vi "Apply Amplitude Envelope.vi"(5 "profile":enum16{"Linear", "Half cosine"}(ring), 6 "time elapsed at transition":dbl, 8 "error in (no error)":errorcluster, 9 "duration":dbl=-1.0, 10 "amplitude modulation":cluster{"start":dbl, "stop":dbl}={"start"=1.0, "stop"=1.0}, 11 "waveform in":waveform(dbl)={"t0"=timestamp(0 s since 1904-01-01), "dt"=0.1, "Y"=[1.0, 1.0, 1.0, 1.0, 1.0]}) -> (0 "error out":errorcluster, 2 "amplitude envelope last value":dbl, 3 "waveform out":waveform(dbl)={"t0"=timestamp(0 s since 1904-01-01), "dt"=nan, "Y"=[]})   [LabVIEW 2017, in "SV Signal.lvclass"]
uses:
  <vilib>/addons/_NISVFA/_Generation/Signal Generation/SV Signal/SV Signal.lvclass
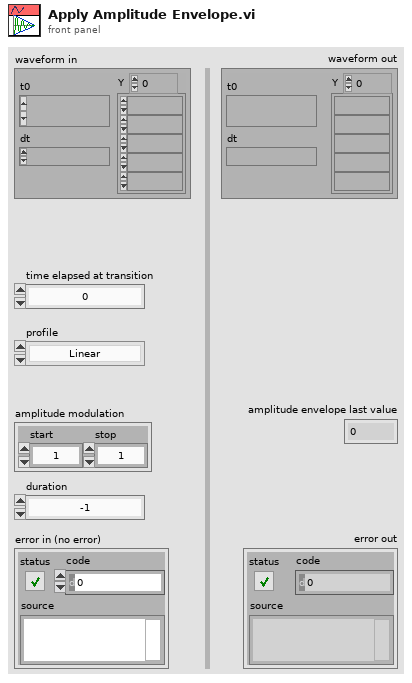
[diagram p1: front panel]
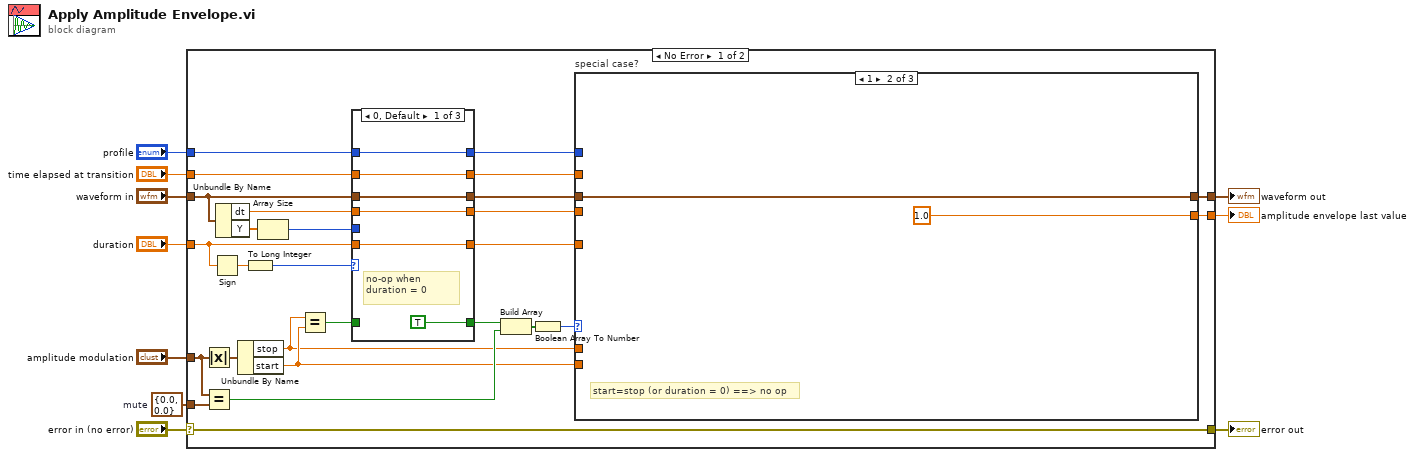
[diagram p0: block diagram]
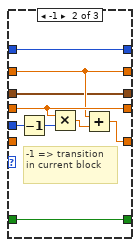
[diagram p2: hidden frame]
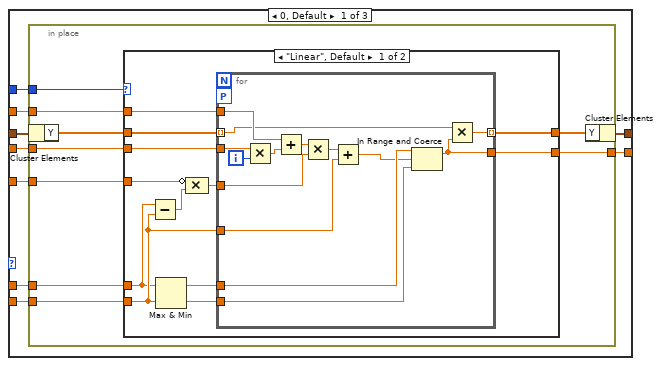
[diagram p4: hidden frame]
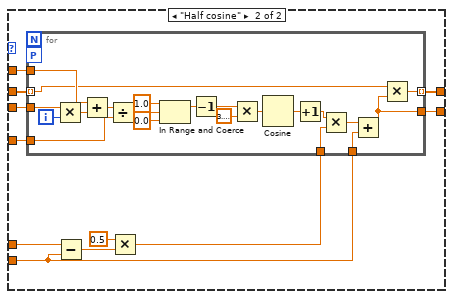
[diagram p5: hidden frame]
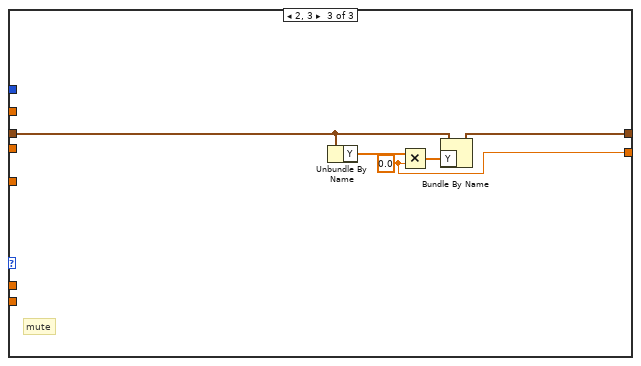
[diagram p6: hidden frame]
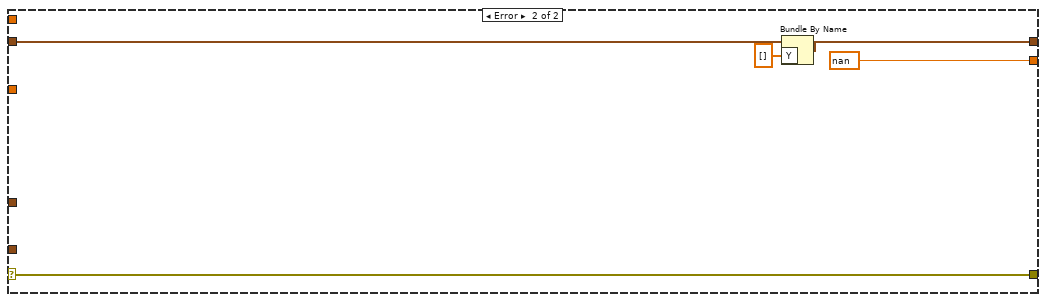
[diagram p7: hidden frame]
diagram:
  w6 = cluster{"start":dbl, "stop":dbl} {"start"=0.0, "stop"=0.0}  # mute
  n1 = case shown="No Error" "error in (no error)" {
    selector: "error in (no error)" -> [w13 w144]
    tunnel: "amplitude modulation" -> [w37 _]
    tunnel: [w36 nan ("start")] -> w9
    tunnel: "time elapsed at transition" -> [w22 _]
    tunnel: "profile" -> [w24 _]
    tunnel: w6 -> [w29 _]
    tunnel: "duration" -> [w19 _]
    tunnel: [w28 w142] -> w4
    tunnel: "waveform in" -> [w18 w143]
    tunnel: [w13 w144] -> w1
    frame No Error {
      n2 = Absolute Value(x=w37) -> (abs(x)=w30:cluster{"start":dbl, "stop":dbl})
      n3 = Equal?(x=w37, y=w29) -> (x = y?=w33:bool)
      n4 = Sign(1:w19) -> (0:w27:dbl)
      n5 = Unbundle By Name(w18) -> ("dt"=w15:dbl, "Y"=w17:dbl[])
      n6 = Unbundle By Name(w30) -> ("stop"=w31:dbl, "start"=w32:dbl)
      n7 = To Long Integer(number=w27) -> (32bit integer=w26:i32)
      n8 = Array Size(array=w17) -> (size(s)=w16:i32)
      n9 = Equal?(x=w31, y=w32) -> (x = y?=w12:bool)
      n10 = case shown="0, Default" w26 {
        tunnel: [w43 w52 w58] -> w25
        tunnel: w24 -> [w43 w52 w58]
        tunnel: [w42 w49 w57] -> w23
        tunnel: w22 -> [w42 w49 w57]
        tunnel: [w41 w46 w56] -> w21
        tunnel: w18 -> [w41 w46 w56]
        tunnel: [w40 w47 w55] -> w20
        tunnel: w19 -> [w40 _ w55]
        tunnel: w16 -> [_ w51 _]
        tunnel: w15 -> [w39 w50 w54]
        tunnel: [w39 w50 w54] -> w14
        tunnel: w12 -> [_ w44 w53]
        tunnel: [TRUE w44 w53] -> w11
        frame 0, Default {
          # "no-op when duration = 0"
        }
        frame -1 {
          # "-1 => transition in current block"
          n11 = Decrement(x=w51) -> (x-1=w45:i32)
          n12 = Multiply(x=w50, y=w45) -> (x*y=w48:dbl)
          n13 = Add(x=w49, y=w48) -> (x+y=w47:dbl)
        }
        frame 1 {
        }
      }
      n14 = Build Array(w11, w33) -> (w34:bool[])
      n15 = Boolean Array To Number(Boolean array=w34) -> (number=w35:u32)
      n16 = case "special case?" shown="1" w35 {
        tunnel: w21 -> [w67 w136 w138]
        tunnel: [w66 w136 w141] -> w28
        tunnel: w20 -> [w65 _ _]
        tunnel: w31 -> [w62 _ _]
        tunnel: w32 -> [w61 _ _]
        tunnel: w25 -> [w64 _ _]
        tunnel: w23 -> [w63 _ _]
        tunnel: w14 -> [w60 _ _]
        tunnel: [w59 1.0 ("t") w137] -> w36
        frame 0, Default {
          n17 = in-place {
            in-place-border: w63 -> [w74]
            in-place-border: w64 -> [w70]
            in-place-border: w65 -> [w73]
            in-place-border: w62 -> [w69]
            in-place-border: w61 -> [w68]
            in-place-border: w60 -> [w72]
            in-place-border: [w71] -> w59
            n18 = in-place-cluster #1(w67) -> ("Y"=w76:dbl[])
            n19 = case shown="\"Linear\", Default" w70 {
              tunnel: w76 -> [w88 w113]
              tunnel: w72 -> [w87 w112]
              tunnel: w74 -> [w86 w107]
              tunnel: [w85 w111] -> w75
              tunnel: w73 -> [w81 w110]
              tunnel: w68 -> [w79 w104]
              tunnel: [w80 w106] -> w71
              tunnel: w69 -> [w78 w105]
              frame "Linear", Default {
                n20 = Subtract(x=w78, y=w79) -> (x-y=w77:dbl)
                n21 = Max & Min(x=w78, y=w79) -> (max(x,y)=w84:dbl, min(x,y)=w83:dbl)
                n22 = Compound Arithmetic op=MULTIPLY(invert w81, w77) -> (w82:dbl)
                n23 = for {
                  tunnel: w88 -> [w99] mode=indexing
                  tunnel: w87 -> [w102]
                  tunnel: w86 -> [w100]
                  tunnel: [w98] -> w85 mode=indexing
                  tunnel: w82 -> [w97]
                  tunnel: w79 -> [w95]
                  tunnel: w84 -> [w92]
                  tunnel: w83 -> [w91]
                  tunnel: [w90] -> w80
                  workers-P: _ -> [_]
                  i -> [w93]
                  n24 = Multiply(x=w102, y=w93) -> (x*y=w101:dbl)
                  n25 = Add(x=w100, y=w101) -> (x+y=w96:dbl)
                  n26 = Multiply(x=w96, y=w97) -> (x*y=w94:dbl)
                  n27 = Add(x=w94, y=w95) -> (x+y=w89:dbl)
                  n28 = In Range and Coerce(upper limit=w92, x=w89, lower limit=w91) -> (coerced(x)=w90:dbl)  [unwired: 1 out]
                  n29 = Multiply(x=w99, y=w90) -> (x*y=w98:dbl)
                }
              }
              frame "Half cosine" {
                n30 = Subtract(x=w105, y=w104) -> (x-y=w103:dbl)
                n31 = Multiply(x=0.5 ("y"), y=w103) -> (x*y=w108:dbl)
                n32 = for {
                  tunnel: w113 -> [w131] mode=indexing
                  tunnel: w112 -> [w134]
                  tunnel: w107 -> [w132]
                  tunnel: [w130] -> w111 mode=indexing
                  tunnel: w110 -> [w128]
                  tunnel: w108 -> [w117]
                  tunnel: w104 -> [w116]
                  tunnel: [w114] -> w106
                  workers-P: _ -> [_]
                  i -> [w127]
                  n33 = Multiply(x=w134, y=w127) -> (x*y=w133:dbl)
                  n34 = Add(x=w132, y=w133) -> (x+y=w129:dbl)
                  n35 = Divide(x=w129, y=w128) -> (x/y=w125:dbl)
                  n36 = In Range and Coerce(upper limit=1.0, x=w125, lower limit=0.0) -> (coerced(x)=w124:dbl)  [unwired: 1 out]
                  n37 = Decrement(x=w124) -> (x-1=w122:dbl)
                  n38 = Multiply(x=w122, y=3.141592653589793) -> (x*y=w121:dbl)
                  n39 = Cosine(x=w121) -> (cos(x)=w119:dbl)
                  n40 = Increment(x=w119) -> (x+1=w115:dbl)
                  n41 = Multiply(x=w115, y=w117) -> (x*y=w118:dbl)
                  n42 = Add(x=w118, y=w116) -> (x+y=w114:dbl)
                  n43 = Multiply(x=w131, y=w114) -> (x*y=w130:dbl)
                }
              }
            }
            n44 = in-place-cluster #1("Y"=w75) -> (w66:waveform(dbl))
          }
        }
        frame 1 {
          # "start=stop (or duration = 0) ==> no op"
        }
        frame 2, 3 {
          w137 = 0.0 ("start")
          # "mute"
          n45 = Unbundle By Name(w138) -> ("Y"=w140:dbl[])
          n46 = Multiply(x=w140, y=w137) -> (x*y=w139:dbl[])
          n47 = Bundle By Name(cluster=w138, "Y"=w139) -> (w141:waveform(dbl))
        }
      }
    }
    frame Error {
      n48 = Bundle By Name(cluster=w143, "Y"=dbl[] []) -> (w142:waveform(dbl))
    }
  }
  "amplitude envelope last value" <- w9
  "waveform out" <- w4
  "error out" <- w1
